vi "Wrap Or Recurse.vi"(7 "Actor in":refnum<class "Actor.lvclass">, 8 "Error in":errorcluster, 10 "Msg DVR in":refnum<data-value>) -> (0 "Error out":errorcluster, 2 "Msg DVR out":refnum<data-value>, 5 "Actor out":refnum<class "Actor.lvclass">)   [LabVIEW 2020, in "jettl.lvlib"]
uses:
  jettl.lvlib
  Msg/Msg.lvclass
  Actor/Actor.lvclass
  Refs/Refs.lvclass
  Unified Actor Relation.ctl
  Teller.ctl
  Msg.ctl
  Msg Contents/Msg Contents.lvclass
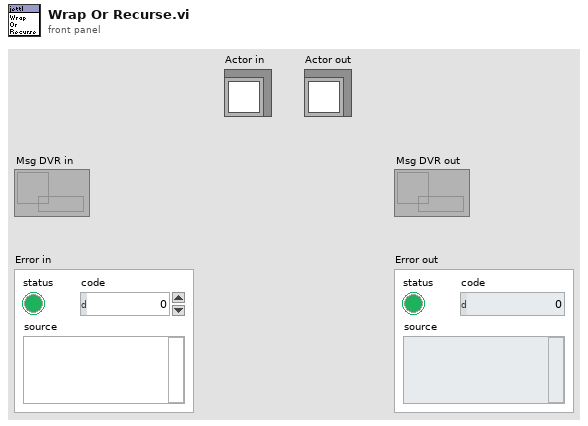
[diagram p1: front panel]
types:
  T1 = typedef "jettl.lvlib/Msg.ctl" = cluster{"Msg":refnum<class "Msg.lvclass">, "Msg Contents":refnum<class "Msg Contents.lvclass">, "Teller":T2}
  T2 = typedef "jettl.lvlib/Teller.ctl" = cluster{"Unified Actor Alias":string, "Unified Actor Relation":T3, "Absolute Time":timestamp, "Relative Time":dbl}
  T3 = typedef "jettl.lvlib/Unified Actor Relation.ctl" = enum16{"Self", "Parent", "Child"}
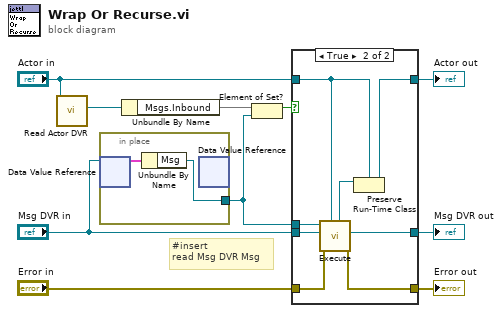
[diagram p0: block diagram]
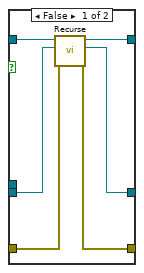
[diagram p2: hidden frame]
diagram:
  # "#insert\nread Msg DVR Msg"
  n1 = call-dynamic "Read Actor DVR.vi"("Actor in"="Actor in") -> ("Actor DVR"=w5:refnum<data-value>)  [unwired: 10 in]
  n2 = in-place {
    in-place-border: [w11] -> w1
    n3 = in-place-dvr #1("Msg DVR in") -> (w12:T1)  [unwired: 1 out]
    n4 = Unbundle By Name(w12) -> ("Msg"=w11:refnum<class "Msg.lvclass">)
    n5 = in-place-dvr #1() -> ()  [unwired: 1 in, 2 out]
  }
  n6 = Unbundle By Name(w5) -> ("Msgs.Inbound"=w4)
  n7 = Element of Set?(10:w1, 11:w4) -> (3:w8:bool)
  n8 = case shown="True" w8 {
    tunnel: "Actor in" -> [w16 w23]
    tunnel: [w17 w22] -> w9
    tunnel: "Msg DVR in" -> [w14 w20]
    tunnel: [w18 w26] -> w10
    tunnel: [w13 w19] -> w3
    tunnel: "Error in" -> [w15 w25]
    tunnel: w1 -> [_ w21]
    frame False {
      n9 = call-dynamic "Recurse.vi"("Error in"=w15, "Msg DVR in"=w14, "Actor in"=w16) -> ("Error out"=w18:errorcluster, "Msg DVR out"=w13:refnum<data-value>, "Actor out"=w17:refnum<class "Actor.lvclass">)  [unwired: 6 in]
    }
    frame True {
      n10 = call-dynamic "Execute.vi"("Actor in"=w23, "Error in"=w25, "Msg DVR in"=w20, "Msg in"=w21) -> ("Error out"=w26:errorcluster, "Msg DVR out"=w19:refnum<data-value>, "Actor out"=w24:refnum<class "Actor.lvclass">)  [unwired: 5 in]
      n11 = Preserve Run-Time Class(object in=w24, 2:w23) -> (object out=w22:refnum<class "Actor.lvclass">)  [unwired: 1 in, 1 out]
    }
  }
  "Error out" <- w10
  "Actor out" <- w9
  "Msg DVR out" <- w3
